vi "擦除flash.vi"(8 "error in":errorcluster, 9 "dwLen":u32, 10 "dwAddr":u32) -> (0 "error out":errorcluster)   [LabVIEW 2016]
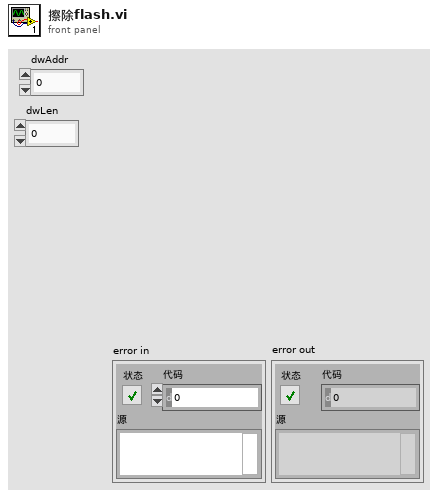
[diagram p1: front panel]
types:
  T1 = cluster{"byCmdType":u8, "bySubCmd":u8, "byPara":u8, "byAddr_h":u8, "byAddr_l":u8, "byAddr_ll":u8, "byLen_h":u8, "byLen_l":u8}
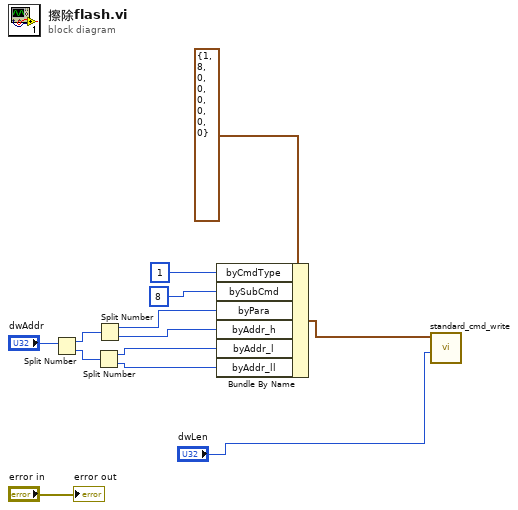
[diagram p0: block diagram]
diagram:
  n1 = Split Number(x="dwAddr") -> (hi(x)=w9:u16, lo(x)=w8:u16)
  n2 = Split Number(x=w8) -> (hi(x)=w5:u8, lo(x)=w4:u8)
  n3 = Split Number(x=w9) -> (hi(x)=w7:u8, lo(x)=w6:u8)
  n4 = Bundle By Name(cluster=T1 {"byCmdType"=1, "bySubCmd"=8, "byPara"=0, "byAddr_h"=0, "byAddr_l"=0, "byAddr_ll"=0, "byLen_h"=0, "byLen_l"=0} ("cmd_std_header_t"), "byCmdType"=u8 1, "bySubCmd"=u8 8, "byPara"=w7, "byAddr_h"=w6, "byAddr_l"=w5, "byAddr_ll"=w4) -> (w3:T1)
  n5 = call "standard_cmd_write.vi"("dwLen"="dwLen", "cmd_std_header_t"=w3) -> ()  [unwired: 9 in, 1 out]
  "error out" <- "error in"
